vi "Duplicate.vi"(8 "error in":errorcluster, 10 "parameters":variant, 11 "node in":refnum<class "NISE_CEF_serializable node.lvclass">) -> (0 "error out":errorcluster, 3 "node copy out":refnum<class "NISE_CEF_serializable node.lvclass">)   [LabVIEW 2013, in "NISE_CEF_serializable node.lvclass"]
doc: "Implements the specific behavior of a node when it is being duplicated\nCan be used to change the name of the new node for example adding Copy to it."
uses:
  NISE_CEF_serializable node.lvclass
  serializable configuration/NISE_CEF_serializable configuration.lvclass
  Write configuration.vi
  Read configuration.vi
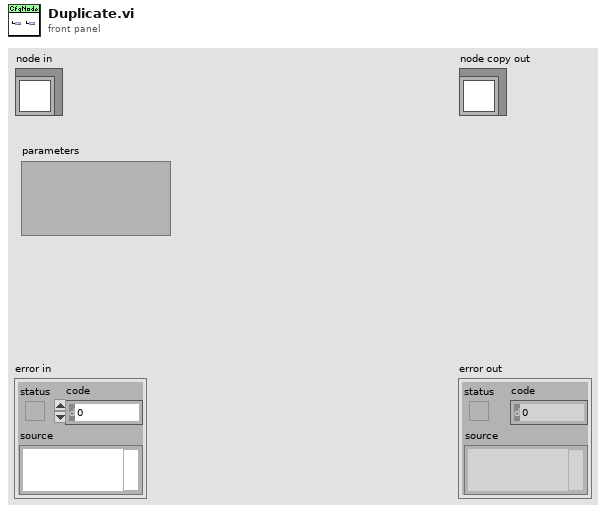
[diagram p1: front panel]
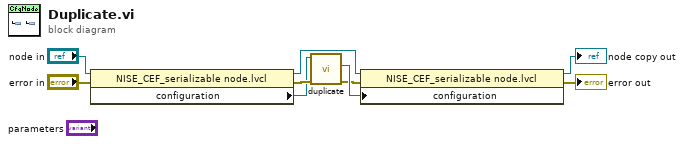
[diagram p0: block diagram]
diagram:
  n1 = property class="NISE_CEF_serializable node.lvcl"(reference="node in", error in="error in") -> (reference out=w3:refnum<class "NISE_CEF_serializable node.lvclass">, error out=w5:errorcluster, "configuration"=w4:refnum<class "NISE_CEF_serializable configuration.lvclass">)
  n2 = call-dynamic "duplicate.vi"("error in"=w5, "configuration in"=w4) -> ("error out"=w1:errorcluster, "duplicate configuration out"=w2:refnum<class "NISE_CEF_serializable configuration.lvclass">)  [unwired: 7 in, 1 out]
  n3 = property class="NISE_CEF_serializable node.lvcl"(reference=w3, error in=w1, "configuration"=w2) -> (reference out=→"node copy out":refnum<class "NISE_CEF_serializable node.lvclass">, error out=→"error out":errorcluster)
